vi "ReadMercuryVISA_Bfield.vi"() -> ()   [LabVIEW 2014]
panel:
  out "Numeric 2":dbl
  out "String Full":string
  out "Numeric":dbl
  out "error out":errorcluster
  in  "error in (no error)":errorcluster
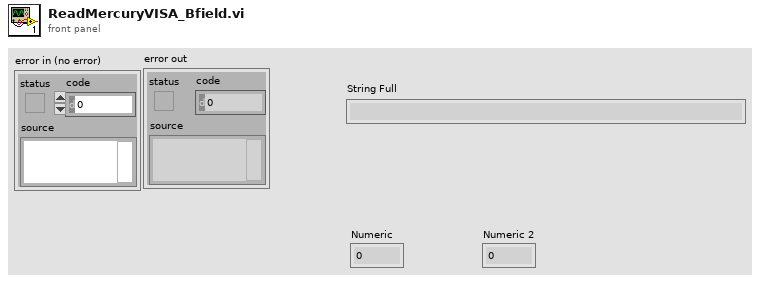
[diagram p1: front panel]
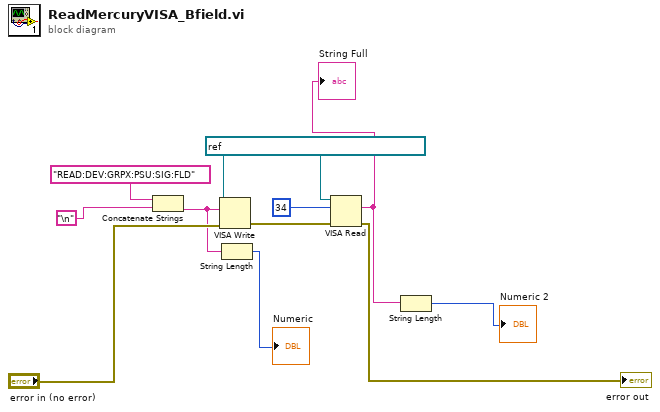
[diagram p0: block diagram]
diagram:
  w9 = refnum<visa-resource-name> "TCPIP0::192.168.128.3::7020::SOCKET" ("VISA resource name")
  n1 = Concatenate Strings("READ:DEV:GRPX:PSU:SIG:FLD" ("string"), "\n") -> (w5:string)
  n2 = VISA Write(VISA resource name=w9, write buffer=w5, error in (no error)="error in (no error)") -> (error out=w10:errorcluster)  [unwired: 2 out]
  n3 = String Length(string=w5) -> (length=→"Numeric":i32)
  n4 = VISA Read(VISA resource name=w9, byte count=34, error in (no error)=w10) -> (read buffer=w2:string, error out=→"error out":errorcluster)  [unwired: 2 out]
  "String Full" <- w2
  n5 = String Length(string=w2) -> (length=→"Numeric 2":i32)
